vi "Select motor.vi"(8 "error in (no error)":errorcluster, 11 "ICS in":refnum<class "ICS.lvclass">) -> (0 "error out":errorcluster, 1 "valid":bool, 2 "selected motor":refnum<class "Motor.lvclass">, 3 "ICS out":refnum<class "ICS.lvclass">)   [LabVIEW 2018, in "ICS.lvclass"]
uses:
  ICS.lvclass
  Motor/Motor.lvclass
  ICS.lvclass/ICS.ctl
  StateManager/StateManager.lvclass/StateManager.ctl
  MotorManager/MotorManager.lvclass
  C:/Dados/SPARC4/Automacao 2022/S4ICS/StateManager/StateManager.lvclass
  StateManager/StateManager.lvclass
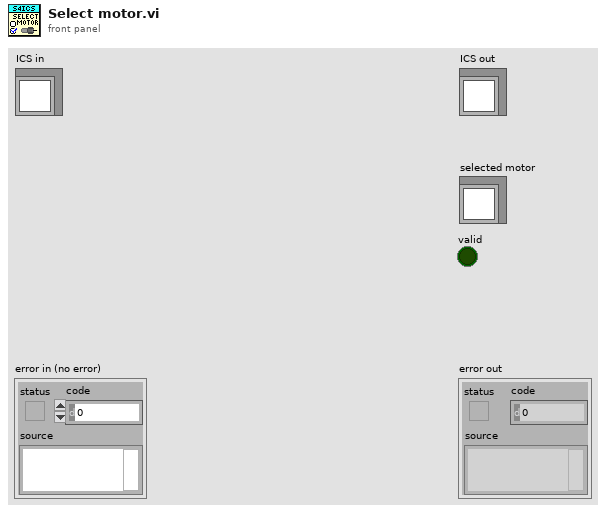
[diagram p1: front panel]
types:
  T1 = cluster{"mode":string, "condition":string, "position":string, "pos_name":string, "pos_id":string}
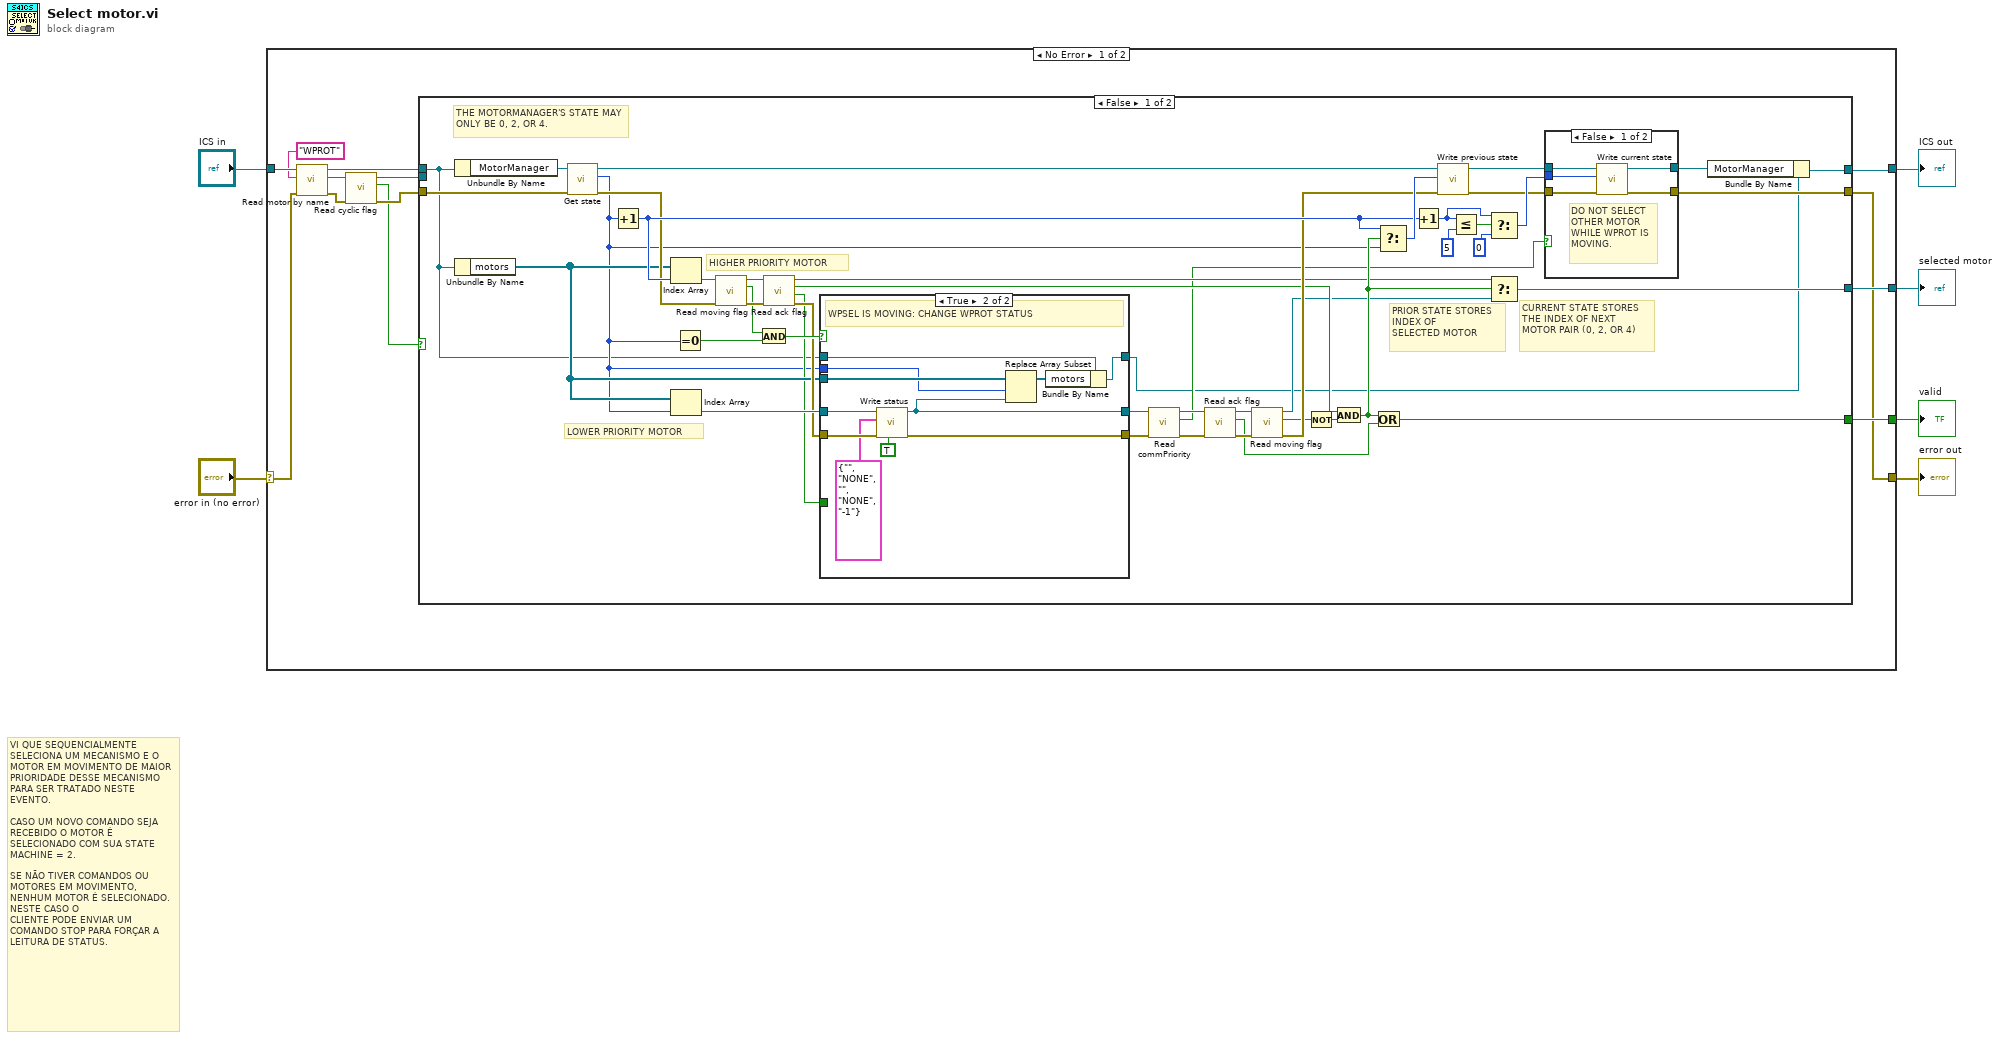
[diagram p0: block diagram]
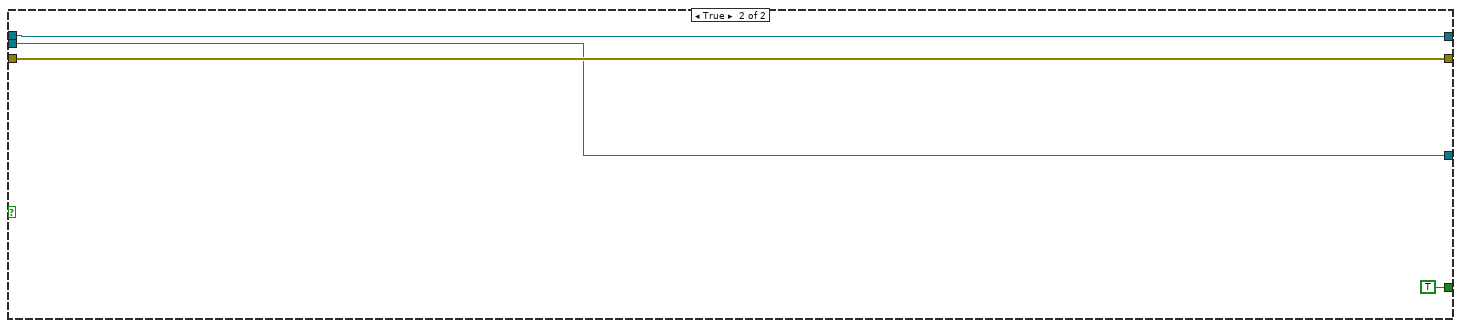
[diagram p4: hidden frame]
diagram:
  # "VI QUE SEQUENCIALMENTE SELECIONA UM MECANISMO E O MOTOR EM MOVIMENTO DE MAIOR PRIORIDADE DESSE MECANISMO PARA SER TRATADO NESTE EVENTO. \n\nCASO UM NOVO COMANDO SEJA RECEBIDO O MOTOR É SELECIONADO COM SUA STATE MACHINE = 2. \n\nSE NÃO TIVER COMANDOS OU MOTORES EM MOVIMENTO, NENHUM MOTOR É SELECIONADO.  NESTE CASO O\nCLIENTE PODE ENVIAR UM COMANDO STOP PARA FORÇAR A LEITURA DE STATUS."
  n1 = case shown="No Error" "error in (no error)" {
    selector: "error in (no error)" -> [w14 w91]
    tunnel: [w17 w91] -> w5
    tunnel: [w7 w92] -> w3
    tunnel: "ICS in" -> [w16 w92]
    tunnel: [w19 _] -> w2
    tunnel: [w18 _] -> w1
    frame No Error {
      n2 = call-dynamic "Read motor by name.vi"("error in (no error)"=w14, "motor name"="WPROT", "ICS in"=w16) -> ("error out"=w11:errorcluster, "Motor.lvclass"=w12:refnum<class "Motor.lvclass">, "ICS out"=w13:refnum<class "ICS.lvclass">)  [unwired: 5 in, 1 out]
      n3 = call-dynamic "Read cyclic flag.vi"("error in (no error)"=w11, "Motor in"=w12) -> ("error out"=w10:errorcluster, "cyclic"=w9:bool, "Motor out"=w8:refnum<class "Motor.lvclass">)  [unwired: 7 in]
      n4 = case shown="False" w9 {
        tunnel: [w61 TRUE] -> w19
        tunnel: [w60 w88] -> w18
        tunnel: [w59 w89] -> w17
        tunnel: w13 -> [w20 w90]
        tunnel: w10 -> [w24 w89]
        tunnel: w8 -> [_ w88]
        tunnel: [w21 w90] -> w7
        frame False {
          # "CURRENT STATE STORES \nTHE INDEX OF NEXT \nMOTOR PAIR (0, 2, OR 4)"
          # "PRIOR STATE STORES\nINDEX OF \nSELECTED MOTOR"
          # "LOWER PRIORITY MOTOR"
          # "HIGHER PRIORITY MOTOR"
          # "THE MOTORMANAGER'S STATE MAY ONLY BE 0, 2, OR 4."
          n5 = Unbundle By Name(w20) -> ("MotorManager"=w54:refnum<class "MotorManager.lvclass">)
          n6 = Unbundle By Name(w20) -> ("motors"=w35:refnum<class "Motor.lvclass">[])
          n7 = call "Get state.vi"("error in (no error)"=w24, "StateManager in"=w54) -> ("error out"=w43:errorcluster, "currentState"=w33:u32, "StateManager out"=w57:refnum<class "MotorManager.lvclass">)  [unwired: 4 in, 3 out]
          n8 = Increment(x=w33) -> (x+1=w51:u32)
          n9 = Index Array(array=w35, index=w51) -> (element=w44:refnum<class "Motor.lvclass">)
          n10 = Index Array(array=w35, index=w33) -> (element=w38:refnum<class "Motor.lvclass">)
          n11 = Equal To 0?(x=w33) -> (x = 0?=w31:bool)
          n12 = call-dynamic "Read moving flag.vi"("error in (no error)"=w43, "Motor in"=w44) -> ("error out"=w41:errorcluster, "moving"=w40:bool, "Motor out"=w42:refnum<class "Motor.lvclass">)  [unwired: 7 in]
          n13 = And(x=w40, y=w31) -> (x .and. y?=w39:bool)
          n14 = call-dynamic "Read ack flag.vi"("error in (no error)"=w41, "Motor in"=w42) -> ("error out"=w37:errorcluster, "stop"=w34:bool, "ack"=w47:bool, "Motor out"=w36:refnum<class "Motor.lvclass">)  [unwired: 6 in]
          n15 = case shown="True" w39 {
            tunnel: w38 -> [w74 w86]
            tunnel: [w74 w79] -> w30
            tunnel: w37 -> [w75 w85]
            tunnel: [w75 w78] -> w28
            tunnel: w20 -> [w73 w80]
            tunnel: w35 -> [_ w83]
            tunnel: w33 -> [_ w82]
            tunnel: [w73 w77] -> w23
            tunnel: w34 -> [_ _]
            frame False {
              # "WPSEL IS NOT MOVING OR OTHER MECHANISM"
            }
            frame True {
              # "WPSEL IS MOVING: CHANGE WPROT STATUS"
              n16 = call-dynamic "Write status.vi"("hold if empty"=TRUE, "error in (no error)"=w85, "status"=T1 {"mode"="", "condition"="NONE", "position"="", "pos_name"="NONE", "pos_id"="-1"}, "Motor in"=w86) -> ("error out"=w78:errorcluster, "Motor out"=w79:refnum<class "Motor.lvclass">)  [unwired: 6 in]
              n17 = Replace Array Subset(array=w83, new element=w79, index=w82) -> (w81:refnum<class "Motor.lvclass">[])
              n18 = Bundle By Name(cluster=w80, "motors"=w81) -> (w77:refnum<class "ICS.lvclass">)
            }
          }
          n19 = call-dynamic "Read commPriority.vi"("error in (no error)"=w28, "Motor in"=w30) -> ("error out"=w27:errorcluster, "commPriority"=w26:bool, "Motor out"=w29:refnum<class "Motor.lvclass">)  [unwired: 7 in]
          n20 = call-dynamic "Read ack flag.vi"("error in (no error)"=w27, "Motor in"=w29) -> ("error out"=w50:errorcluster, "ack"=w46:bool, "Motor out"=w48:refnum<class "Motor.lvclass">)  [unwired: 6 in, 1 out]
          n21 = call-dynamic "Read moving flag.vi"("error in (no error)"=w50, "Motor in"=w48) -> ("error out"=w49:errorcluster, "moving"=w32:bool, "Motor out"=w25:refnum<class "Motor.lvclass">)  [unwired: 7 in]
          n22 = Not(x=w32) -> (.not. x?=w52:bool)
          n23 = And(x=w47, y=w52) -> (x .and. y?=w45:bool)
          n24 = Or(x=w45, y=w46) -> (x .or. y?=w61:bool)
          n25 = Select(t=w51, s=w45, f=w33) -> (s? t:f=w53:u32)
          n26 = Increment(x=w51) -> (x+1=w65:u32)
          n27 = call-dynamic "Write previous state.vi"("error in (no error)"=w49, "previousState"=w53, "StateManager in"=w57) -> ("error out"=w56:errorcluster, "StateManager out"=w55:refnum<class "MotorManager.lvclass">)  [unwired: 7 in]
          n28 = Less Or Equal?(x=w65, y=u32 5) -> (x <= y?=w64:bool)
          n29 = Select(t=w65, s=w64, f=u32 0) -> (s? t:f=w58:u32)
          n30 = Select(t=w36, s=w45, f=w25) -> (s? t:f=w60:refnum<class "Motor.lvclass">)
          n31 = case shown="False" w26 {
            tunnel: [w70 w71] -> w59
            tunnel: w58 -> [w69 _]
            tunnel: w56 -> [w68 w71]
            tunnel: w55 -> [w67 w72]
            tunnel: [w66 w72] -> w22
            frame False {
              # "DO NOT SELECT OTHER MOTOR\nWHILE WPROT IS MOVING."
              n32 = call-dynamic "Write current state.vi"("error in (no error)"=w68, "currentState"=w69, "StateManager in"=w67) -> ("error out"=w70:errorcluster, "StateManager out"=w66:refnum<class "MotorManager.lvclass">)  [unwired: 7 in]
            }
            frame True {
            }
          }
          n33 = Bundle By Name(cluster=w23, "MotorManager"=w22) -> (w21:refnum<class "ICS.lvclass">)
        }
        frame True {
        }
      }
    }
    frame Error {
    }
  }
  "error out" <- w5
  "ICS out" <- w3
  "valid" <- w2
  "selected motor" <- w1
